vi "Delay.vi"(8 "error in (no error)":errorcluster, 10 "Delay (ms)":u32, 11 "VISA resource name":refnum<visa-resource-name>) -> (0 "error out":errorcluster, 3 "VISA resource name out":refnum<visa-resource-name>)   [LabVIEW 2015, in "RIGOL DS1000 Series.lvlib"]
doc: "Delay before sending commands to instrument."
uses:
  RIGOL DS1000 Series.lvlib
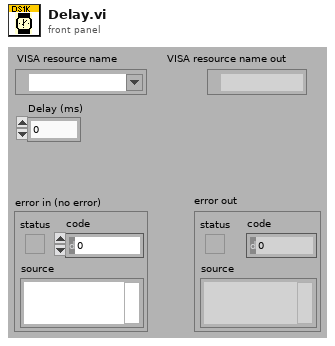
[diagram p1: front panel]
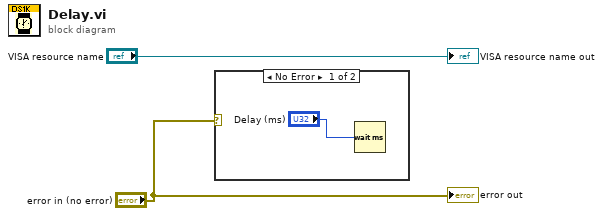
[diagram p0: block diagram]
diagram:
  n1 = case shown="No Error" "error in (no error)" {
    frame No Error {
      n2 = Wait (ms)(milliseconds to wait="Delay (ms)") -> ()  [unwired: 1 out]
    }
    frame Error {
    }
  }
  "VISA resource name out" <- "VISA resource name"
  "error out" <- "error in (no error)"
